vi "c ctre phoenixpro deserialize bool.vi"(7 "val":bool, 8 "error in (no error)":errorcluster, 9 "strlen":u32, 10 "str":string, 11 "spn":i32) -> (0 "error out":errorcluster, 3 "function return":i32, 5 "val out":bool)   [LabVIEW 2020, in "CTRE_PhoenixTools.lvlib"]
doc: "CTREXPORT int c_ctre_phoenixpro_deserialize_bool(int spn, const char *str, uint32_t strlen, bool *val);"
uses:
  <userlib>/CTRE_PhoenixTools/CTRE_PhoenixTools.lvlib
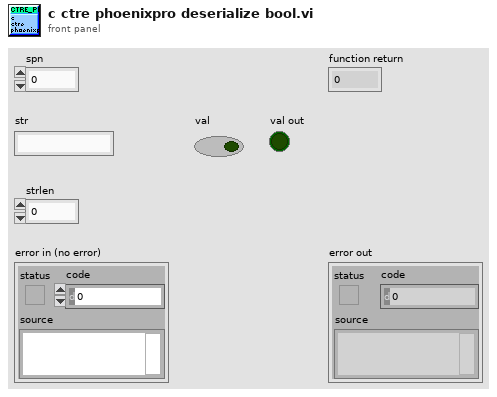
[diagram p1: front panel]
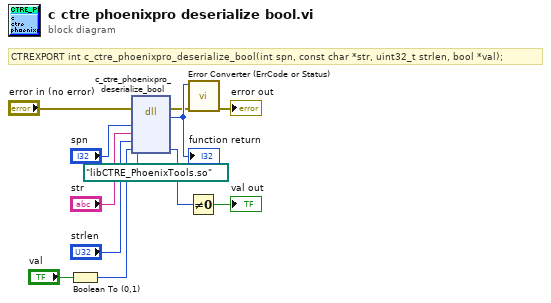
[diagram p0: block diagram]
diagram:
  # "CTREXPORT int c_ctre_phoenixpro_deserialize_bool(int spn, const char *str, uint32_t strlen, bool *val);"
  n1 = Boolean To (0,1)(Boolean="val") -> (0, 1=w7:i16)
  n2 = dll-call lib="?" fn="c_ctre_phoenixpro_deserialize_bool"(path in=path "libCTRE_PhoenixTools.so", error in="error in (no error)", "spn"="spn", "str"="str", "strlen"="strlen", "val"=w7) -> (error out=w3:errorcluster, w12:i32, "val"=w5:u8)  [unwired: 4 in, 1 out]
  "function return" <- w12
  n3 = Not Equal To 0?(x=w5) -> (x != 0?=→"val out":bool)
  n4 = call <userlib>:"Error Converter (ErrCode or Status).vi"("error in (no error)"=w3, "error code"=w12) -> ("error out"=→"error out":errorcluster)  [unwired: 9 in]
